vi "Read Cells for Errors.vi"(8 "error in (no error)":errorcluster, 10 "Error Cells (ex:A12)":string[](array[string]), 11 "NI_report in":refnum<class "NI_report.lvclass">) -> (0 "error out":errorcluster, 1 "Pass?":bool, 2 "Error Code":i32, 3 "NI_report out":refnum<class "NI_report.lvclass">)   [LabVIEW 2015]
uses:
  <vilib>/Utility/NIReport.llb/NI_report.lvclass
  <vilib>/addons/_office/excel.llb/Excel Get Data (str).vi
  <vilib>/addons/_office/NI_ReportGenerationToolkit.lvlib
  <vilib>/Utility/NIReport.llb/Excel/NI_Excel.lvclass
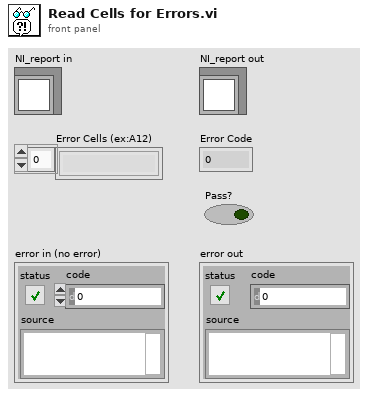
[diagram p1: front panel]
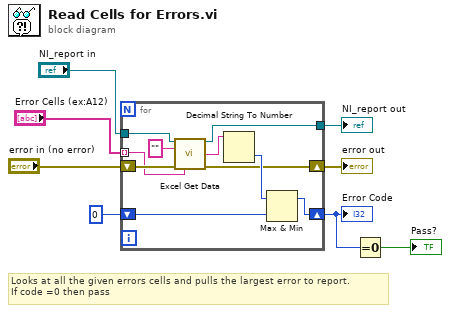
[diagram p0: block diagram]
diagram:
  # "Looks at all the given errors cells and pulls the largest error to report. \nIf code =0 then pass"
  n1 = for {
    tunnel: "NI_report in" -> [w18]
    tunnel: "Error Cells (ex:A12)" -> [w15] mode=indexing
    tunnel: [w14] -> w7
    shift-right: [w10] -> w5
    shift-left: 0 -> [w13]
    shift-right: [w9] -> w8
    shift-left: "error in (no error)" -> [w16]
    n2 = call-poly <vilib>:"Excel Get Data.vi"("report in"=w18, "data type"="", "error in (no error)"=w16, "name (\"\")"=w15) -> ("report out"=w14:refnum<class "NI_report.lvclass">, "data"=w12:string, "error out"=w9:errorcluster)  [unwired: 9 in]
    n3 = Decimal String To Number(string=w12) -> (number=w11:i32)  [unwired: 2 in, 1 out]
    n4 = Max & Min(x=w11, y=w13) -> (max(x,y)=w10:i32)  [unwired: 1 out]
  }
  "error out" <- w8
  "NI_report out" <- w7
  "Error Code" <- w5
  n5 = Equal To 0?(x=w5) -> (x = 0?=→"Pass?":bool)
